vi "RSS Logon.vi"(6 "RSS Operation":T2(ring), 8 "error in (no error)":errorcluster, 9 "Password":string, 10 "Logon User":string, 11 "Domain":string) -> (0 "error out":errorcluster, 1 "standard output":string, 2 "Active Dir. Info":T1, 3 "Logon OK":bool)   [LabVIEW 2020]
uses:
  Control/Active Dir Info.ctl
  <vilib>/Utility/error.llb/whitespace.ctl
panel:
  out "RSSLogon Path":path
  out "Username":string
  out "Hostname":string
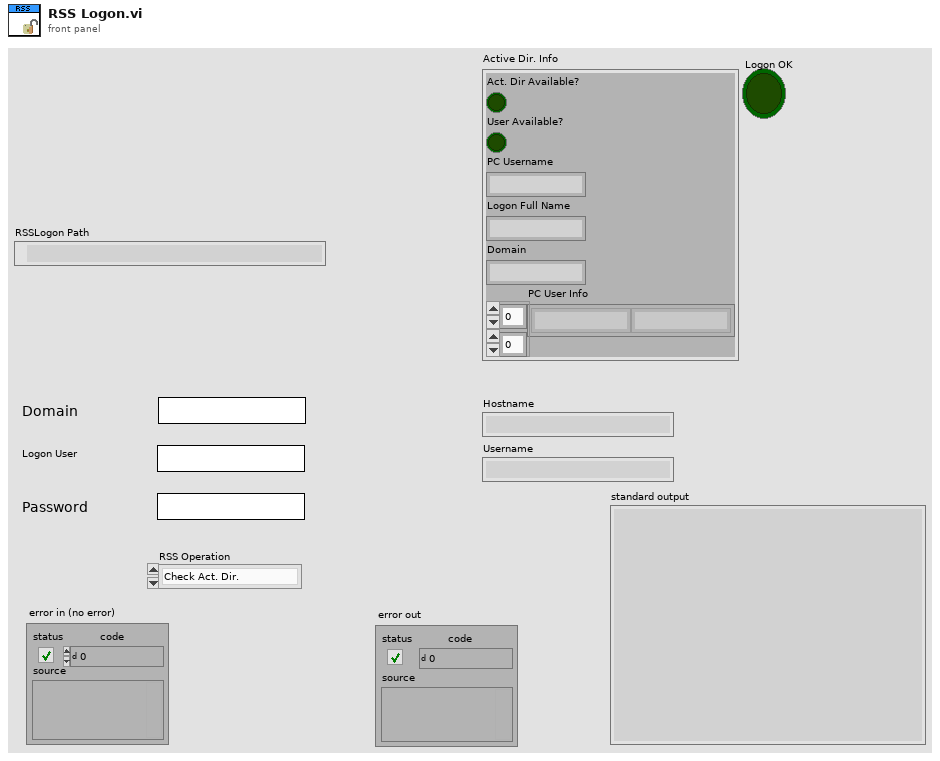
[diagram p1: front panel]
types:
  T1 = typedef "Active Dir Info.ctl" = cluster{"Act. Dir Available?":bool, "User Available?":bool, "PC Username":string, "Logon Full Name":string, "Domain":string, "PC User Info":string[][]}
  T2 = enum16{"Check Act. Dir.", "Logon", "PC User", "PC User Info", "Hostname"}
  T3 = enum32{"invalid app kind", "Development System", "Run Time System", "Student Edition", "Embedded LabVIEW", "Evaluation", "Custom"}
  T4 = typedef "whitespace.ctl" = u16
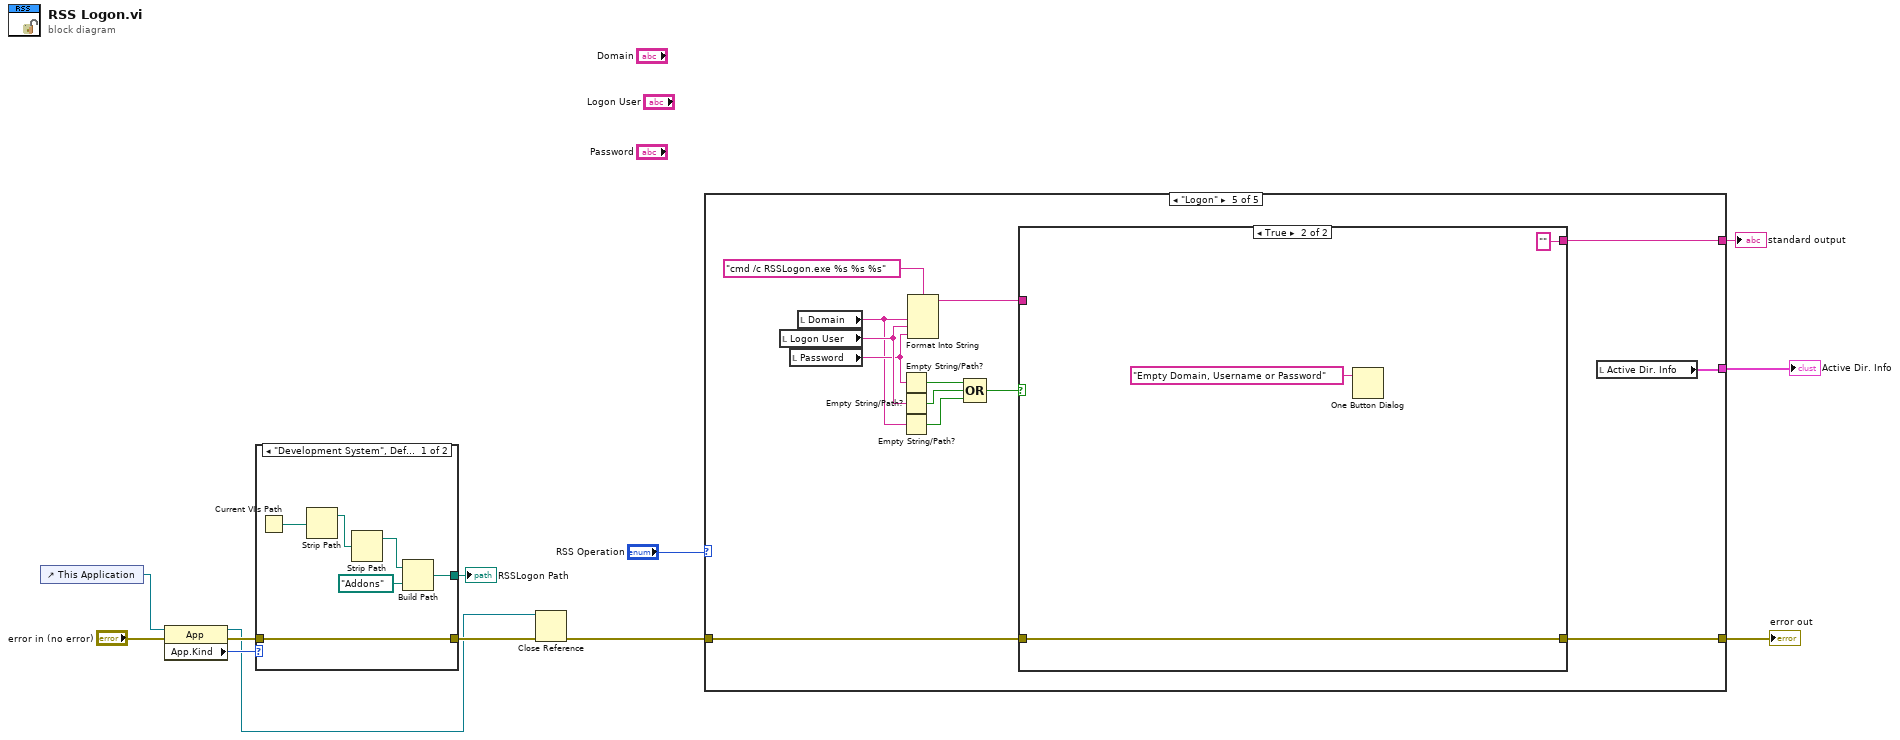
[diagram p0: block diagram]
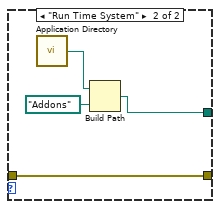
[diagram p2: hidden frame]
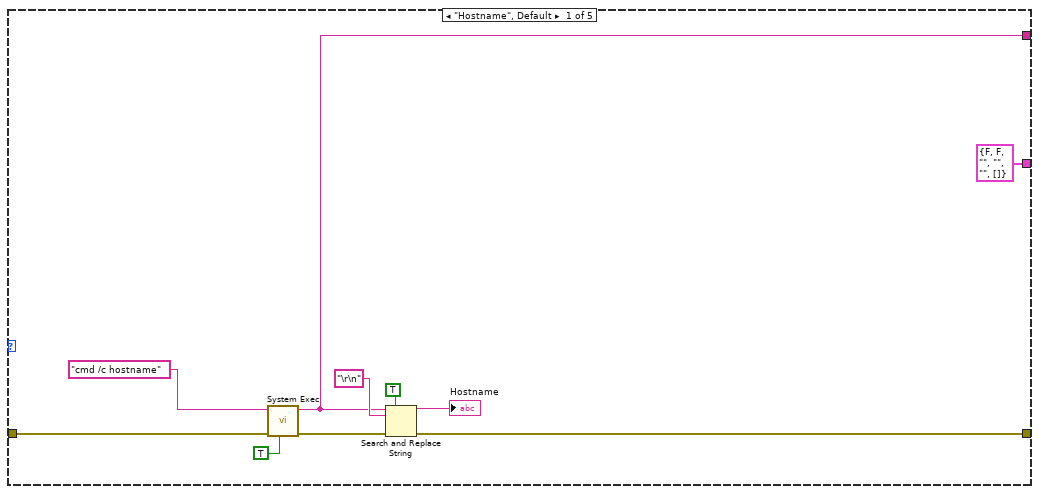
[diagram p3: hidden frame]
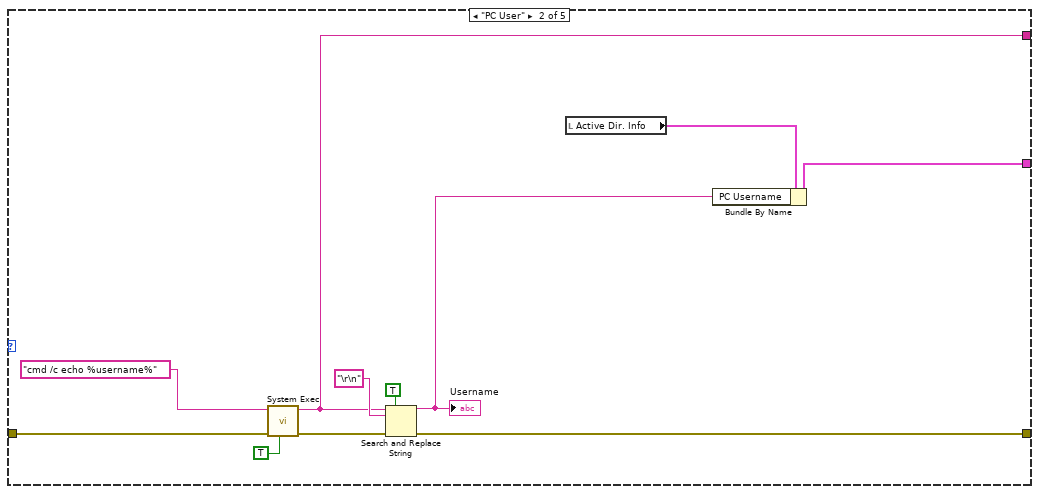
[diagram p4: hidden frame]
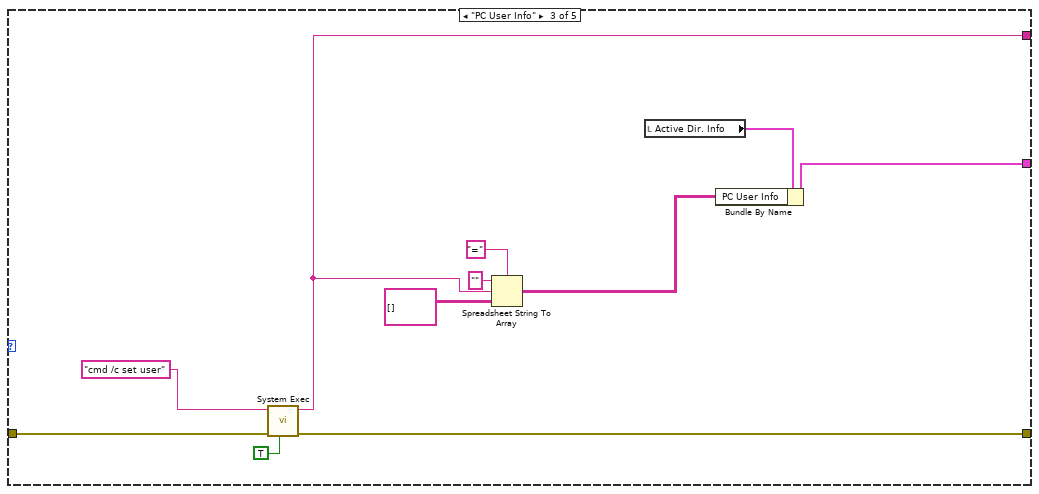
[diagram p5: hidden frame]
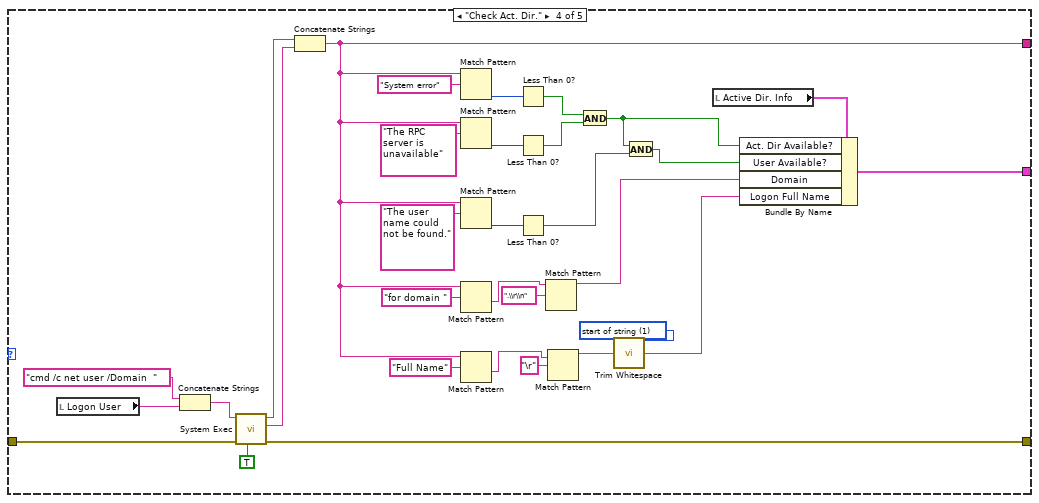
[diagram p6: hidden frame]
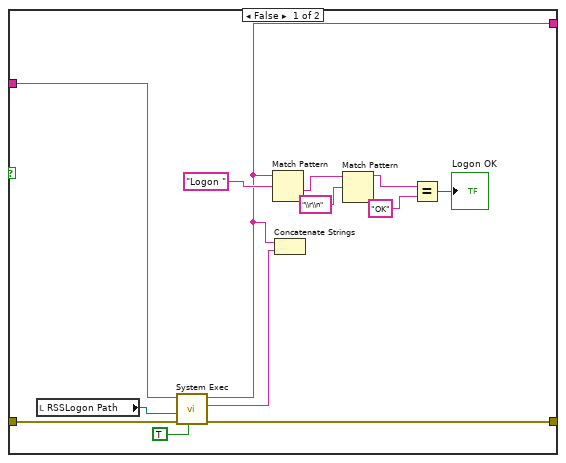
[diagram p7: hidden frame]
diagram:
  n1 = control-ref of="This Application"() -> (w8:refnum<vi>)
  n2 = property class="App"(reference=w8, error in="error in (no error)") -> (reference out=w1:refnum<vi>, error out=w5:errorcluster, "App.Kind"=w6:T3)
  n3 = case shown="\"Development System\", Default" w6 {
    tunnel: w5 -> [w18 w19]
    tunnel: [w18 w19] -> w3
    tunnel: [w13 w20] -> w4
    frame "Development System", Default {
      n4 = Current VI's Path() -> (path=w17:path)
      n5 = Strip Path(path=w17) -> (stripped path=w16:path)  [unwired: 1 out]
      n6 = Strip Path(path=w16) -> (stripped path=w15:path)  [unwired: 1 out]
      n7 = Build Path(base path=w15, name or relative path=path "Addons") -> (appended path=w13:path)
    }
    frame "Run Time System" {
      n8 = call <vilib>:"Application Directory.vi"() -> ("Application Directory"=w22:path)
      n9 = Build Path(base path=w22, name or relative path=path "Addons") -> (appended path=w20:path)
    }
  }
  "RSSLogon Path" <- w4
  n10 = Close Reference(reference=w1, error in (no error)=w3) -> (error out=w2:errorcluster)
  n11 = case shown="\"Logon\"" "RSS Operation" {
    tunnel: w2 -> [w30 w41 w52 w85 w99]
    tunnel: [w25 w37 w51 w84 w88] -> w11
    tunnel: [w24 w36 w50 w69 w89] -> w10
    tunnel: [T1 {"Act. Dir Available?"=FALSE, "User Available?"=FALSE, "PC Username"="", "Logon Full Name"="", "Domain"="", "PC User Info"=[]} ("Active Dir. Info") w35 w49 w60 w87] -> w9
    frame "Hostname", Default {
      n12 = call <vilib>:"System Exec.vi"("run minimized? (F)"=TRUE, "error in (no error)"=w30, "command line"="cmd /c hostname") -> ("error out"=w27:errorcluster, "standard output"=w24:string)  [unwired: 5 in, 2 out]
      n13 = Search and Replace String(replace all?=TRUE ("replace all? (F)"), input string=w24, search string="\r\n", error in=w27) -> (result string=→"Hostname":string, error out=w25:errorcluster)  [unwired: 4 in, 2 out]
    }
    frame "PC User" {
      n14 = call <vilib>:"System Exec.vi"("run minimized? (F)"=TRUE, "error in (no error)"=w41, "command line"="cmd /c echo %username%") -> ("error out"=w38:errorcluster, "standard output"=w36:string)  [unwired: 5 in, 2 out]
      n15 = Search and Replace String(replace all?=TRUE ("replace all? (F)"), input string=w36, search string="\r\n", error in=w38) -> (result string=w34:string, error out=w37:errorcluster)  [unwired: 4 in, 2 out]
      "Username" <- w34
      n16 = local read "Active Dir. Info"() -> (w33:T1)
      n17 = Bundle By Name(cluster=w33, "PC Username"=w34) -> (w35:T1)
    }
    frame "PC User Info" {
      n18 = call <vilib>:"System Exec.vi"("run minimized? (F)"=TRUE, "error in (no error)"=w52, "command line"="cmd /c set user") -> ("error out"=w51:errorcluster, "standard output"=w50:string)  [unwired: 5 in, 2 out]
      n19 = Spreadsheet String To Array(delimiter (Tab)="=", format string="", spreadsheet string=w50, array type (2D Dbl)=string[][] [] ("PC User Info")) -> (array=w46:string[][])
      n20 = local read "Active Dir. Info"() -> (w44:T1)
      n21 = Bundle By Name(cluster=w44, "PC User Info"=w46) -> (w49:T1)
    }
    frame "Check Act. Dir." {
      w65 = T4 1 items=["both", "start of string", "end of string"] ("location (both)")
      n22 = local read "Logon User"() -> (w56:string)
      n23 = Concatenate Strings("cmd /c net user /Domain  " ("command line"), w56) -> (w82:string)
      n24 = call <vilib>:"System Exec.vi"("run minimized? (F)"=TRUE, "error in (no error)"=w85, "command line"=w82) -> ("error out"=w84:errorcluster, "standard error"=w80:string, "standard output"=w81:string)  [unwired: 5 in, 1 out]
      n25 = Concatenate Strings(w81, w80) -> (w69:string)
      n26 = Match Pattern(string=w69, regular expression="System error") -> (offset past match=w73:i32)  [unwired: 1 in, 3 out]
      n27 = Match Pattern(string=w69, regular expression="The RPC server is unavailable") -> (offset past match=w72:i32)  [unwired: 1 in, 3 out]
      n28 = Match Pattern(string=w69, regular expression="The user name could not be found.") -> (offset past match=w71:i32)  [unwired: 1 in, 3 out]
      n29 = Match Pattern(string=w69, regular expression="for domain ") -> (after substring=w74:string)  [unwired: 1 in, 3 out]
      n30 = Match Pattern(string=w69, regular expression="Full Name") -> (after substring=w67:string)  [unwired: 1 in, 3 out]
      n31 = Less Than 0?(x=w73) -> (x < 0?=w64:bool)
      n32 = Less Than 0?(x=w72) -> (x < 0?=w63:bool)
      n33 = Less Than 0?(x=w71) -> (x < 0?=w57:bool)
      n34 = Match Pattern(string=w74, regular expression=".\\r\\n") -> (before substring=w62:string)  [unwired: 1 in, 3 out]
      n35 = Match Pattern(string=w67, regular expression="\r") -> (before substring=w66:string)  [unwired: 1 in, 3 out]
      n36 = And(x=w64, y=w63) -> (x .and. y?=w58:bool)
      n37 = call <vilib>:"Trim Whitespace.vi"("string"=w66, "location (both)"=w65) -> ("trimmed string"=w61:string)
      n38 = And(x=w58, y=w57) -> (x .and. y?=w59:bool)
      n39 = local read "Active Dir. Info"() -> (w55:T1)
      n40 = Bundle By Name(cluster=w55, "Act. Dir Available?"=w58, "User Available?"=w59, "Domain"=w62, "Logon Full Name"=w61) -> (w60:T1)
    }
    frame "Logon" {
      n41 = local read "Logon User"() -> (w97:string)
      n42 = local read "Password"() -> (w96:string)
      n43 = local read "Domain"() -> (w95:string)
      n44 = Empty String/Path?(string/path=w96) -> (empty?=w94:bool)
      n45 = Empty String/Path?(string/path=w97) -> (empty?=w93:bool)
      n46 = Empty String/Path?(string/path=w95) -> (empty?=w92:bool)
      n47 = Format Into String(format string="cmd /c RSSLogon.exe %s %s %s", w95, w97, w96) -> (resulting string=w90:string)  [unwired: 2 in, 1 out]
      n48 = Compound Arithmetic op=OR(w94, w93, w92) -> (w91:bool)
      n49 = case shown="True" w91 {
        tunnel: w99 -> [w112 w114]
        tunnel: w90 -> [w110 _]
        tunnel: [w101 "" ("standard output")] -> w89
        tunnel: [w100 w114] -> w88
        frame False {
          n50 = local read "RSSLogon Path"() -> (w111:path)
          n51 = call <vilib>:"System Exec.vi"("run minimized? (F)"=TRUE, "error in (no error)"=w112, "working directory"=w111, "command line"=w110) -> ("error out"=w100:errorcluster, "standard error"=w102:string, "standard output"=w101:string)  [unwired: 4 in, 1 out]
          n52 = Match Pattern(string=w101, regular expression="Logon ") -> (after substring=w107:string)  [unwired: 1 in, 3 out]
          n53 = Concatenate Strings(w101, w102) -> ()  [unwired: 1 out]
          n54 = Match Pattern(string=w107, regular expression="\\r\\n") -> (before substring=w105:string)  [unwired: 1 in, 3 out]
          n55 = Equal?(x=w105, y="OK") -> (x = y?=→"Logon OK":bool)
        }
        frame True {
          n56 = One Button Dialog(message="Empty Domain, Username or Password") -> ()  [unwired: 1 in, 1 out]
        }
      }
      n57 = local read "Active Dir. Info"() -> (w87:T1)
    }
  }
  "error out" <- w11
  "standard output" <- w10
  "Active Dir. Info" <- w9
